vi "CONTROLADOR_DIGITAL_V3.vi"() -> ()   [LabVIEW 2018]
uses:
  <vilib>/MakerHub/LINX/Public/Peripherals/Analog/Analog Read 1 Chan.vi
  <vilib>/MakerHub/LINX/Public/Peripherals/PWM/PWM Set Duty Cycle 1 Chan.vi
  <vilib>/MakerHub/LINX/Public/Peripherals/Analog/Analog Read N Chans.vi
  <vilib>/MakerHub/LINX/Private/Local IO/LinxAnalogRead.vi
  <vilib>/MakerHub/LINX/Public/Utilities/Check Channel.vi
  <vilib>/MakerHub/LINX/Public/Utilities/Open Serial.vi
  <vilib>/MakerHub/LINX/Private/Utilties/Generate Error.vi
  <vilib>/MakerHub/LINX/Public/Peripherals/PWM/PWM Set Duty Cycle N Chans.vi
  <vilib>/MakerHub/LINX/LMH-LINX.lvlib
panel:
  in  "q24":dbl
  in  "q23":dbl
  in  "q22":dbl
  in  "q21":dbl
  in  "q14":dbl
  in  "q13":dbl
  in  "q12":dbl
  in  "q11":dbl
  in  "q04":dbl
  in  "q03":dbl
  in  "q02":dbl
  in  "q01":dbl
  in  "f":dbl
  in  "wk":dbl
  in  "p2":dbl
  in  "p1":dbl
  in  "q1":dbl
  in  "qo":dbl
  in  "Controlador":string(combo)
  in  "time":u32
  out "?":dynamicdata(graph)
  out "uk":dbl
  in  "SP":dbl min=0.0 max=100.0
  out "y":dbl
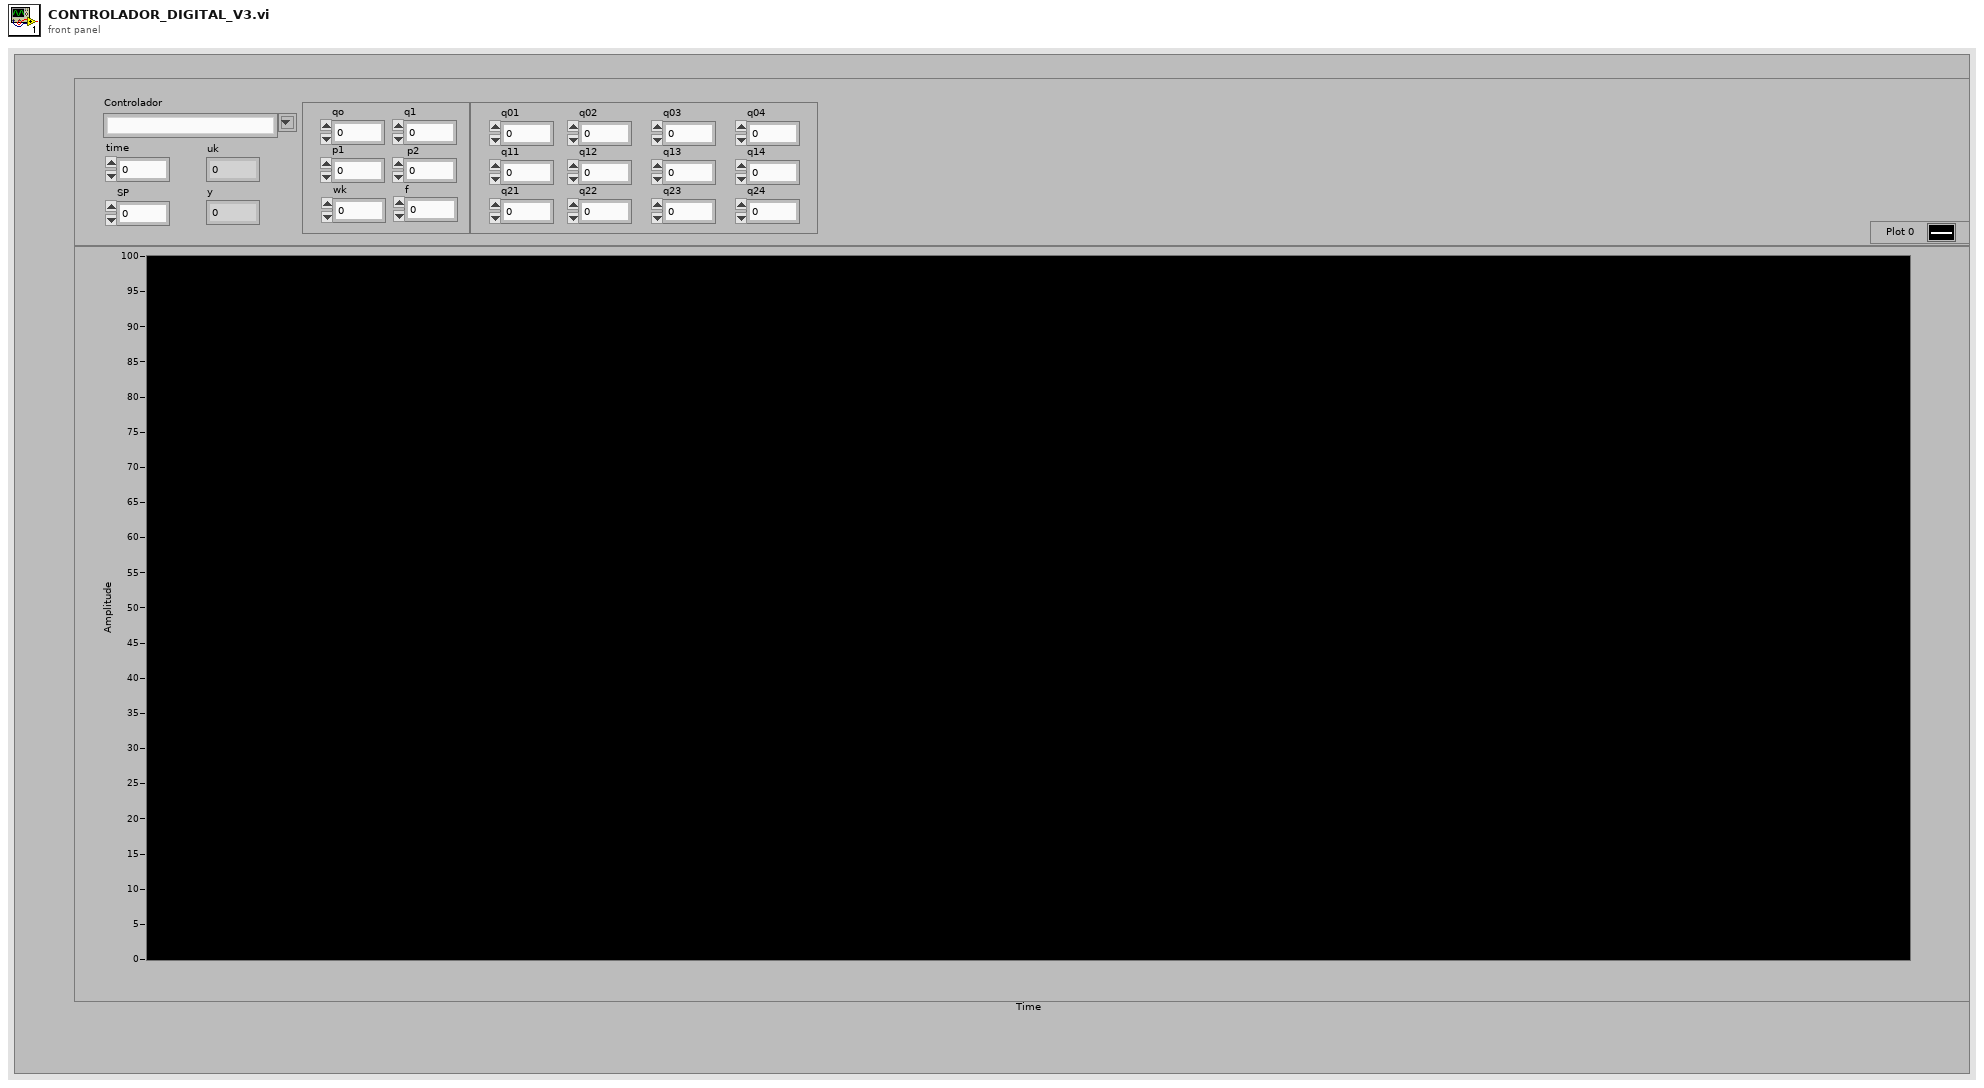
[diagram p1: front panel]
types:
  T1 = typedef "LMH-LINX.lvlib/LINX Ref.ctl" = cluster{"IO":T2, "Interface":T3, "LINX Device Config":T4}
  T2 = typedef "LMH-LINX.lvlib/Platform.ctl" = enum16{"Remote", "Local"}
  T3 = typedef "LMH-LINX.lvlib/Interface.ctl" = enum16{"Serial", "TCP"}
  T4 = typedef "LMH-LINX.lvlib/Device.lvlib/LINX Device Config.ctl" = cluster{"Interface":T3, "COM Port":refnum<visa-resource-name>, "TCP Configuration":T5, "Device Family":u8, "Device ID":u8, "Device Name":string, "TCP Ref":refnum<k5>, "Channels":T6}
  T5 = typedef "LMH-LINX.lvlib/Device.lvlib/TCP Config.ctl" = cluster{"IP Address":string, "Port":u16}
  T6 = typedef "LMH-LINX.lvlib/Channels.ctl" = cluster{"DI":u8[], "DO":u8[], "AI":u8[], "AO":u8[], "PWM":u8[], "QE":u8[], "UART":u8[], "I2C 2":u8[], "SPI":u8[], "CAN":u8[], "Servo":u8[], "AI Ref (V)":dbl, "AI Resolution (Bits)":u8, "AO Ref (V)":dbl, "AO Resolution (Bits)":u8}
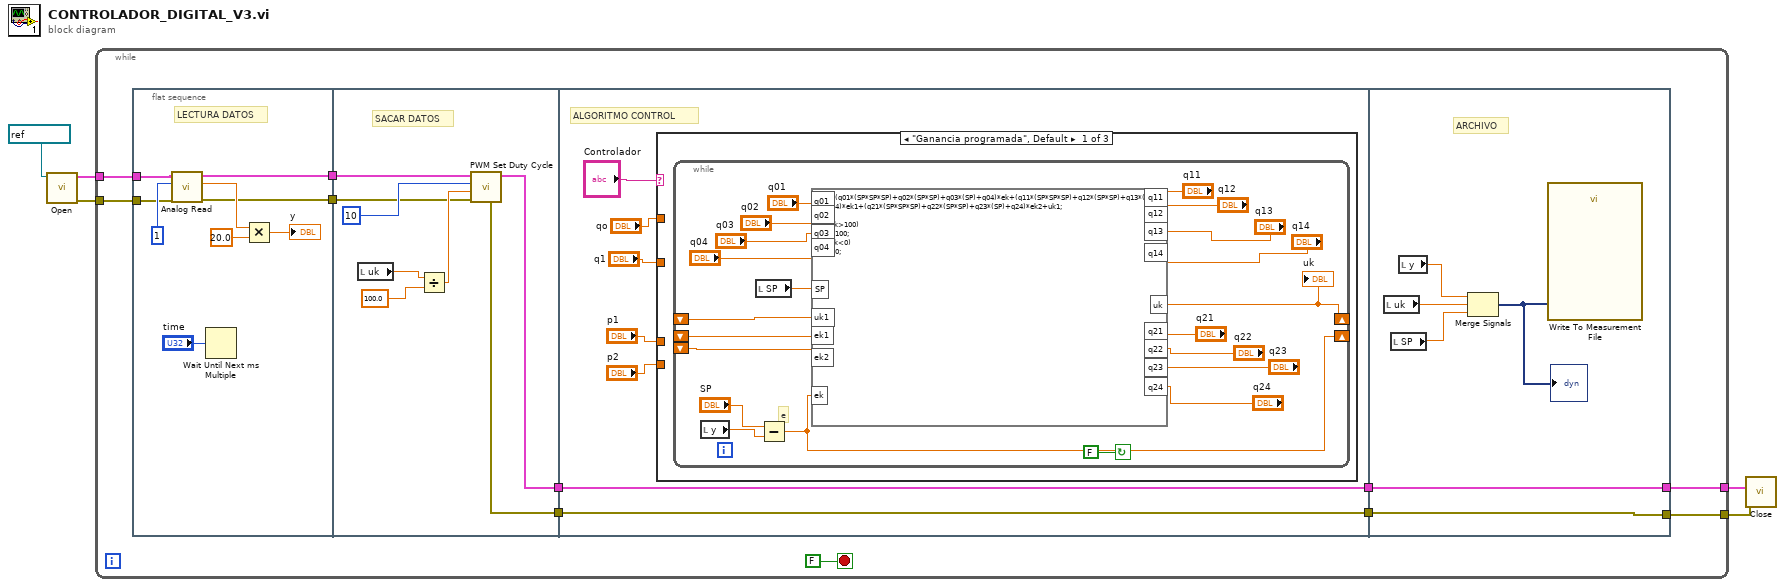
[diagram p0: block diagram]
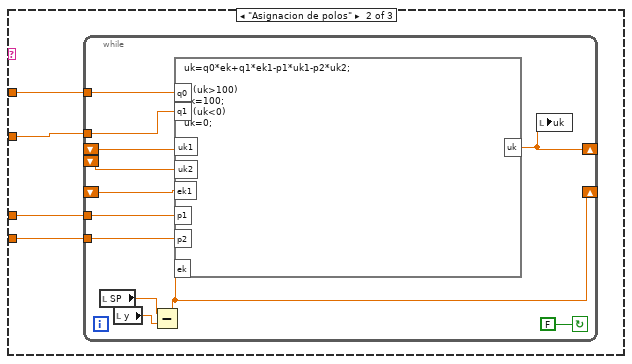
[diagram p2: hidden frame]
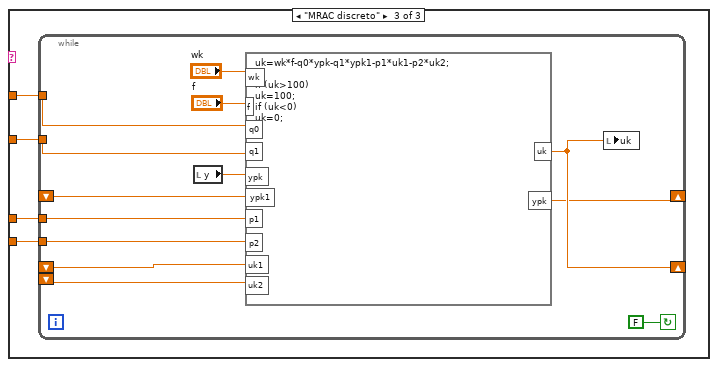
[diagram p3: hidden frame]
diagram:
  n1 = call-poly <vilib>:"Open.vi"("Serial Port"=refnum<visa-resource-name> "COM4") -> ("Error Out"=w3:errorcluster, "LINX Resource"=w5:T1)  [unwired: 8 in, 1 out]
  n2 = while {
    tunnel: w5 -> [w16]
    tunnel: [w14] -> w4
    tunnel: w3 -> [w11]
    tunnel: [w9] -> w2
    stop <- FALSE stop-if-true
    n3 = flat-sequence {
      tunnel: w16 -> [w21]
      tunnel: [w20] -> w15
      tunnel: w11 -> [w19]
      tunnel: [w18] -> w10
      tunnel: w15 -> [w29]
      tunnel: [w28] -> w12
      tunnel: w10 -> [w27]
      tunnel: [w26] -> w7
      tunnel: [w40] -> w13
      tunnel: w12 -> [w40]
      tunnel: [w39] -> w8
      tunnel: w7 -> [w39]
      tunnel: [w96] -> w14
      tunnel: w13 -> [w96]
      tunnel: [w95] -> w9
      tunnel: w8 -> [w95]
      frame #0 {
        # "LECTURA DATOS"
        n4 = call-poly <vilib>:"Analog Read.vi"("Error In"=w19, "Analog Channel"=u8 1, "LINX Resource"=w21) -> ("Error Out"=w18:errorcluster, "Voltage"=w24:dbl, "LINX Resource"=w20:T1)  [unwired: 5 in, 1 out]
        n5 = Wait Until Next ms Multiple(millisecond multiple="time") -> ()  [unwired: 1 out]
        n6 = Multiply(x=w24, y=20.0) -> (x*y=→"y":dbl)
      }
      frame #1 {
        # "SACAR DATOS"
        n7 = local read "uk"() -> (w32:dbl)
        n8 = Divide(x=w32, y=100.0) -> (x/y=w30:dbl)
        n9 = call-poly <vilib>:"PWM Set Duty Cycle.vi"("Error In"=w27, "Duty Cycle (0-1)"=w30, "PWM Channel"=u8 10, "LINX Resource"=w29) -> ("Error Out"=w26:errorcluster, "LINX Resource"=w28:T1)  [unwired: 6 in]
      }
      frame #2 {
        # "ALGORITMO CONTROL"
        n10 = case shown="\"Ganancia programada\", Default" "Controlador" {
          tunnel: "qo" -> [_ w65 w81]
          tunnel: "q1" -> [_ w64 w80]
          tunnel: "p1" -> [_ w63 w79]
          tunnel: "p2" -> [_ w62 w78]
          frame "Ganancia programada", Default {
            n11 = while {
              shift-right: [w46] -> _
              shift-left: _ -> [w59]
              shift-left: _ -> [w58]
              shift-right: [w57] -> _
              shift-left: _ -> [w56]
              stop <- FALSE continue-if-true
              # "e"
              n12 = local read "y"() -> (w60:dbl)
              n13 = local read "SP"() -> (w41:dbl)
              n14 = Subtract(x="SP", y=w60) -> (x-y=w46:dbl)
              n15 = formula code="uk=(q01*(SP*SP*SP)+q02*(SP*SP)+q03*(SP)+q04)*ek+(q11*(SP*SP*SP)+q12*(SP*SP)+q13*(SP)+q14)*ek1+(q21*(SP*SP*SP)+q22*(SP*SP)+q23*(SP)+q24)*ek2+uk1;\n\nif (uk>100)\nuk=100;\nif (uk<0)\nuk=0;"("q01"="q01", "q02"="q02", "q03"="q03", "ek"=w46, "ek1"=w59, "ek2"=w58, "uk1"=w56, "q04"="q04", "q12"="q12", "q13"="q13", "q14"="q14", "q11"="q11", "q21"="q21", "q22"="q22", "q23"="q23", "q24"="q24", "SP"=w41) -> ("uk"=w57:dbl)
              "uk" <- w57
            }
          }
          frame "Asignacion de polos" {
            n16 = while {
              shift-right: [w75] -> _
              shift-left: _ -> [w74]
              shift-right: [w71] -> _
              shift-left: _ -> [w73]
              shift-left: _ -> [w72]
              tunnel: w65 -> [w70]
              tunnel: w64 -> [w69]
              tunnel: w63 -> [w68]
              tunnel: w62 -> [w67]
              stop <- FALSE continue-if-true
              n17 = local read "SP"() -> (w77:dbl)
              n18 = local read "y"() -> (w76:dbl)
              n19 = Subtract(x=w77, y=w76) -> (x-y=w71:dbl)
              n20 = formula code="uk=q0*ek+q1*ek1-p1*uk1-p2*uk2;\n\nif (uk>100)\nuk=100;\nif (uk<0)\nuk=0;"("q0"=w70, "q1"=w69, "uk1"=w74, "ek1"=w73, "uk2"=w72, "ek"=w71, "p1"=w68, "p2"=w67) -> ("uk"=w75:dbl)
              n21 = local write "uk"(w75) -> ()
            }
          }
          frame "MRAC discreto" {
            n22 = while {
              tunnel: w81 -> [w91]
              tunnel: w80 -> [w92]
              tunnel: w79 -> [w90]
              tunnel: w78 -> [w89]
              shift-right: [w88] -> _
              shift-left: _ -> [w87]
              shift-left: _ -> [w86]
              shift-right: [w83] -> _
              shift-left: _ -> [w84]
              stop <- FALSE continue-if-true
              n23 = local read "y"() -> (w85:dbl)
              n24 = formula code="uk=wk*f-q0*ypk-q1*ypk1-p1*uk1-p2*uk2;\n\nif (uk>100)\nuk=100;\nif (uk<0)\nuk=0;"("wk"="wk", "f"="f", "q0"=w91, "q1"=w92, "ypk"=w85, "p1"=w90, "p2"=w89, "uk1"=w87, "uk2"=w86, "ypk1"=w84) -> ("uk"=w88:dbl, "ypk"=w83:dbl)
              n25 = local write "uk"(w88) -> ()
            }
          }
        }
      }
      frame #3 {
        # "ARCHIVO"
        n26 = local read "uk"() -> (w99:dbl)
        n27 = local read "SP"() -> (w98:dbl)
        n28 = local read "y"() -> (w100:dbl)
        n29 = Merge Signals(w100, w99, w98) -> (w97:dynamicdata)
        "?" <- w97
        n30 = call "Write To Measurement File"("Signals"=w97) -> ()  [unwired: 16 in, 3 out]
      }
    }
  }
  n31 = call <vilib>:"Close.vi"("Error In"=w2, "LINX Resource"=w4) -> ()  [unwired: 9 in, 1 out]
